vi "BufferAndScan.vi"(9 "UpdatesPerPoint":u32, 10 "ClockPause":u32=40, 11 "Point Delay(uSec)":u32 caption="Point Delay (uSec)") -> (1 "Sequencing error":bool, 2 "NumRepetitions":i32, 3 "NumPoints":i32)   [LabVIEW 2012]
uses:
  <vilib>/rvi/DataTransferAndStorage/Container/XNode/niFpgaContainer.xnode
  <vilib>/rvi/FIFO/Fifo_Resource/niFpgaFifoEmulationRefIn.vi
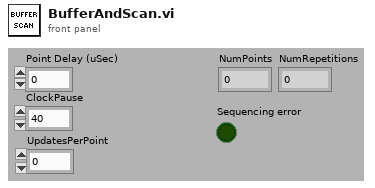
[diagram p1: front panel]
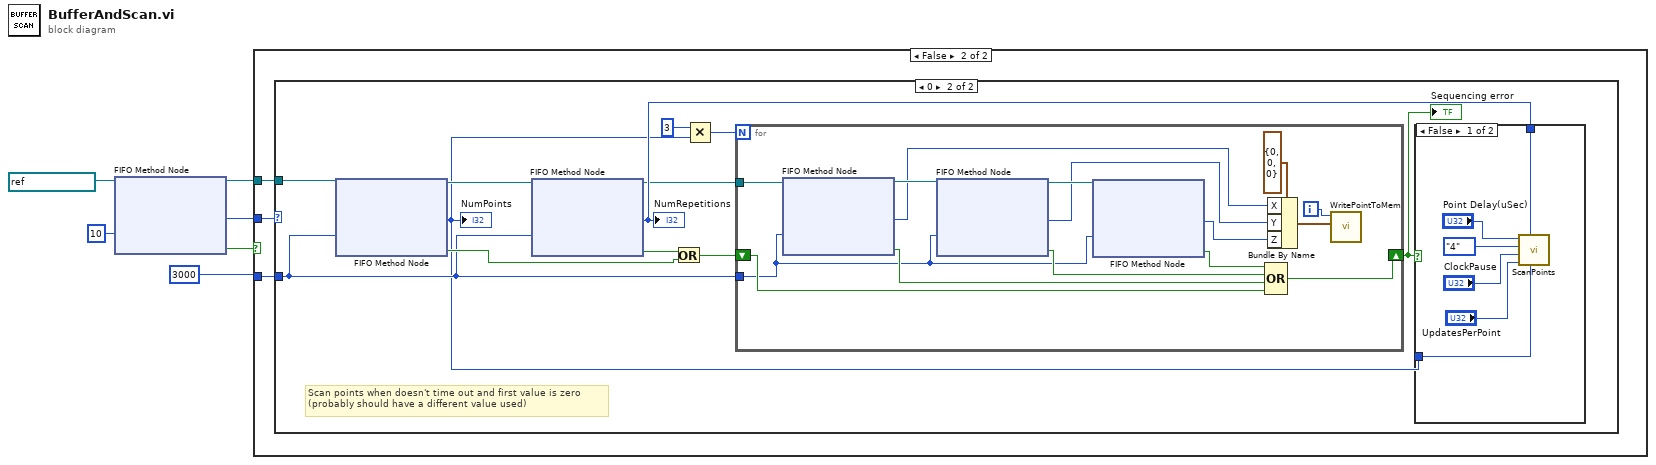
[diagram p0: block diagram]
diagram:
  n1 = xnode ("FIFO Method Node")("Timeout"=10, "FIFO In"=refnum<k21> "Coordinate") -> ("Element"=w4:i32, "Timed Out?"=w3:bool, "FIFO Out"=w5:refnum<k21>)
  n2 = case shown="False" w3 {
    tunnel: w5 -> [_ w9]
    tunnel: w4 -> [_ w8]
    tunnel: 3000 ("Timeout") -> [_ w7]
    frame True {
    }
    frame False {
      n3 = case shown="0" w8 {
        tunnel: w9 -> [_ w20]
        tunnel: w7 -> [_ w14]
        frame Default {
        }
        frame 0 {
          # "Scan points when doesn't time out and first value is zero \n(probably should have a different value used)"
          n4 = xnode ("FIFO Method Node")("Timeout"=w14, "FIFO In"=w20) -> ("Element"=w12:i32, "Timed Out?"=w18:bool, "FIFO Out"=w21:refnum<k21>)
          "NumPoints" <- w12
          n5 = xnode ("FIFO Method Node")("Timeout"=w14, "FIFO In"=w21) -> ("Element"=w13:i32, "Timed Out?"=w19:bool, "FIFO Out"=w11:refnum<k21>)
          "NumRepetitions" <- w13
          n6 = Or(x=w19, y=w18) -> (x .or. y?=w15:bool)
          n7 = Multiply(x=3, y=w12) -> (x*y=w17:i32)
          n8 = for {
            N: w17 -> [_]
            shift-right: [w40] -> w10
            shift-left: w15 -> [w41]
            tunnel: w14 -> [w34]
            tunnel: w11 -> [w39]
            i -> [w28]
            n9 = xnode ("FIFO Method Node")("Timeout"=w34, "FIFO In"=w39) -> ("Element"=w30:i32, "Timed Out?"=w42:bool, "FIFO Out"=w38:refnum<k21>)
            n10 = xnode ("FIFO Method Node")("Timeout"=w34, "FIFO In"=w38) -> ("Element"=w31:i32, "Timed Out?"=w36:bool, "FIFO Out"=w37:refnum<k21>)
            n11 = xnode ("FIFO Method Node")("Timeout"=w34, "FIFO In"=w37) -> ("Element"=w32:i32, "Timed Out?"=w35:bool)  [unwired: 1 out]
            n12 = Compound Arithmetic op=OR(w35, w36, w42, w41) -> (w40:bool)
            n13 = Bundle By Name(cluster=cluster{"X":i32, "Y":i32, "Z":i32} {"X"=0, "Y"=0, "Z"=0} ("Point"), "X"=w30, "Y"=w31, "Z"=w32) -> (w29:cluster{"X":i32, "Y":i32, "Z":i32})
            n14 = call "WritePointToMem.vi"("Point"=w29, "PointNum"=w28) -> ()  [unwired: 10 in]
          }
          "Sequencing error" <- w10
          n15 = case shown="False" w10 {
            tunnel: w13 -> [w27 _]
            tunnel: w12 -> [w26 _]
            frame False {
              n16 = call "ScanPoints.vi"("NumPoints"=w26, "NumberSweeps"=w27, "UpdatesPerPoint"="UpdatesPerPoint", "ClockPause"="ClockPause", "WriteSize"=enum16{"1", "2", "4"}."4", "Point Delay(uSec)"="Point Delay(uSec)") -> ()  [unwired: 6 in]
            }
            frame True {
            }
          }
        }
      }
    }
  }
